vi "TruncI8.vi"(5 "Decimal places":i8, 6 "Number":i8) -> (2 "Truncated number":i8)   [LabVIEW 2017, in "GPNumeric.lvlib"]
doc: "Truncates <B>Number</B> to a number of <B>Decimal places</B>.\n\nSet <B>Decimal places</B> to a negative number to truncate to nearest 10, nearest 100 and so on. E.g. to truncate 782 to the nearest hundred, you set <B>Decimal places</B> to -2 and the <B>Truncated number</B> will be 700.\n\nThis VI is inlined.\n\nSteen Schmidt\nGPower\n16/5 2014"
uses:
  GPNumeric.lvlib
panel:
  # "Copyright © 2014\nGPower\nSee enclosed license file for terms and conditions"
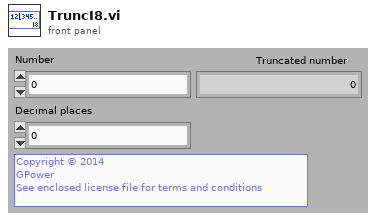
[diagram p1: front panel]
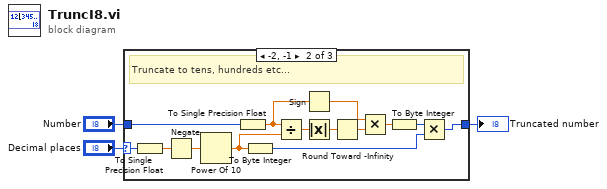
[diagram p0: block diagram]
diagram:
  n1 = case shown="-2, -1" "Decimal places" {
    selector: "Decimal places" -> [_ w14 _]
    tunnel: [_ w11 w18] -> w3
    tunnel: "Number" -> [_ w12 w18]
    frame ..-3 {
      # "Truncate above max value; Return zero."
    }
    frame -2, -1 {
      # "Truncate to tens, hundreds etc..."
      n2 = To Single Precision Float(number=w14) -> (single precision float=w13:sgl)
      n3 = Negate(x=w13) -> (-x=w17:sgl)
      n4 = Power Of 10(x=w17) -> (10^x=w10:sgl)
      n5 = To Single Precision Float(number=w12) -> (single precision float=w5:sgl)
      n6 = To Byte Integer(number=w10) -> (8bit integer=w16:i8)
      n7 = Divide(x=w5, y=w10) -> (x/y=w4:sgl)
      n8 = Sign(1:w5) -> (0:w6:sgl)
      n9 = Absolute Value(x=w4) -> (abs(x)=w9:sgl)
      n10 = Round Toward -Infinity(1:w9) -> (0:w8:sgl)
      n11 = Multiply(x=w6, y=w8) -> (x*y=w7:sgl)
      n12 = To Byte Integer(number=w7) -> (8bit integer=w15:i8)
      n13 = Multiply(x=w15, y=w16) -> (x*y=w11:i8)
    }
    frame 0.. {
      # "Truncate to n decimal places; return integer unchanged."
    }
  }
  "Truncated number" <- w3
